vi "VIQA Control Type Image.vi"(8 "error in (no error)":errorcluster, 11 "VI Refnum":refnum<vi>) -> (0 "error out":errorcluster, 2 "Type Image":T1, 3 "dup VI Refnum":refnum<vi>)   [LabVIEW 2018, in "VI Quality.lvlib"]
doc: "This VI creates a control data type image similar to the context help window display."
uses:
  VI Quality.lvlib
  <vilib>/picture/picture.llb/imagedata.ctl
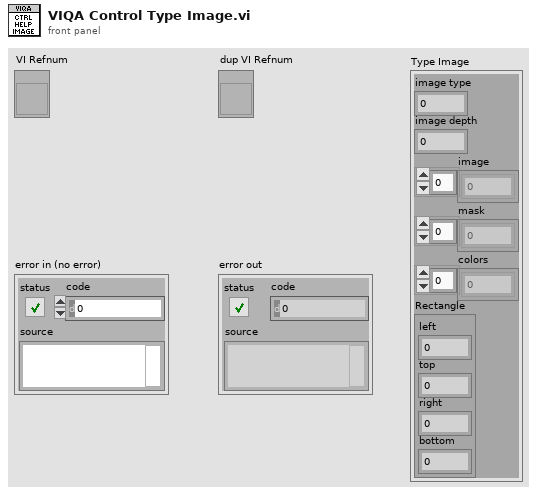
[diagram p1: front panel]
types:
  T1 = typedef "imagedata.ctl" = cluster{"image type":i32, "image depth":i32, "image":u8[], "mask":u8[], "colors":u32[], "Rectangle":cluster{"left":i16, "top":i16, "right":i16, "bottom":i16}}
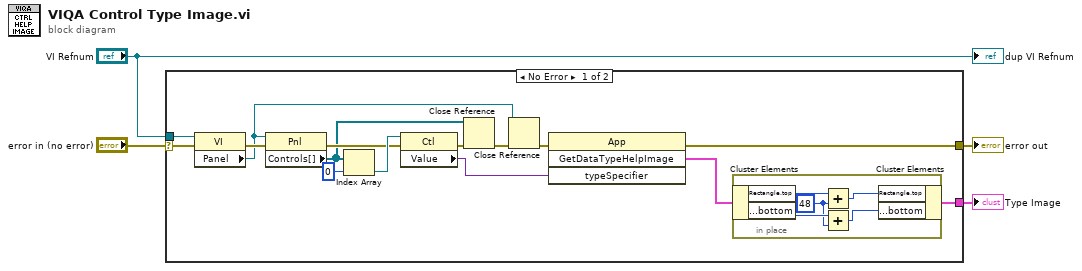
[diagram p0: block diagram]
diagram:
  n1 = case shown="No Error" "error in (no error)" {
    selector: "error in (no error)" -> [w7 w25]
    tunnel: [w8 _] -> w4
    tunnel: [w6 w25] -> w2
    tunnel: "VI Refnum" -> [w5 _]
    frame No Error {
      n2 = property class="VI"(reference=w5, error in=w7) -> (error out=w19:errorcluster, "Panel"=w10:refnum<vi>)  [unwired: 1 out]
      n3 = property class="Pnl"(reference=w10, error in=w19) -> (error out=w16:errorcluster, "Controls[]"=w12:refnum<vi>[])  [unwired: 1 out]
      n4 = Index Array(array=w12, index=0) -> (element=w17:refnum<vi>)
      n5 = property class="Ctl"(reference=w17, error in=w16) -> (error out=w15:errorcluster, "Value"=w14:variant)  [unwired: 1 out]
      n6 = Close Reference(reference=w12, error in (no error)=w15) -> (error out=w11:errorcluster)
      n7 = Close Reference(reference=w10, error in (no error)=w11) -> (error out=w9:errorcluster)
      n8 = invoke class="App" method="GetDataTypeHelpImage"(error in=w9, "typeSpecifier"=w14) -> (error out=w6:errorcluster, "GetDataTypeHelpImage"=w13:T1)  [unwired: 2 in, 2 out]
      n9 = in-place {
        w22 = i16 48 ("y")
        n10 = in-place-cluster #1(w13) -> ("Rectangle.top"=w24:i16, "Rectangle.bottom"=w23:i16)
        n11 = Add(x=w24, y=w22) -> (x+y=w21:i16)
        n12 = Add(x=w23, y=w22) -> (x+y=w20:i16)
        n13 = in-place-cluster #1("Rectangle.top"=w21, "Rectangle.bottom"=w20) -> (w8:T1)
      }
    }
    frame Error {
    }
  }
  "Type Image" <- w4
  "error out" <- w2
  "dup VI Refnum" <- "VI Refnum"
